vi "Disp3D.vi"(1 "Status":enum16{"In", "Out"}(ring)=enum."Out", 2 "MultR":dbl, 3 "TargXYZ":dbl[](array[numeric])=[0.0, 0.0, 0.0], 4 "PosXYZ":dbl[](array[numeric])=[0.0, 0.0, 0.0], 5 "DrawSize":T1, 6 "Blank":picture) -> (0 "Pic":picture)   [LabVIEW 2013]
uses:
  <vilib>/Utility/miscctls.llb/LVBoundsTypeDef.ctl
panel:
  out "DrawSize 2":T1={"Width"=1662, "Height"=1015}
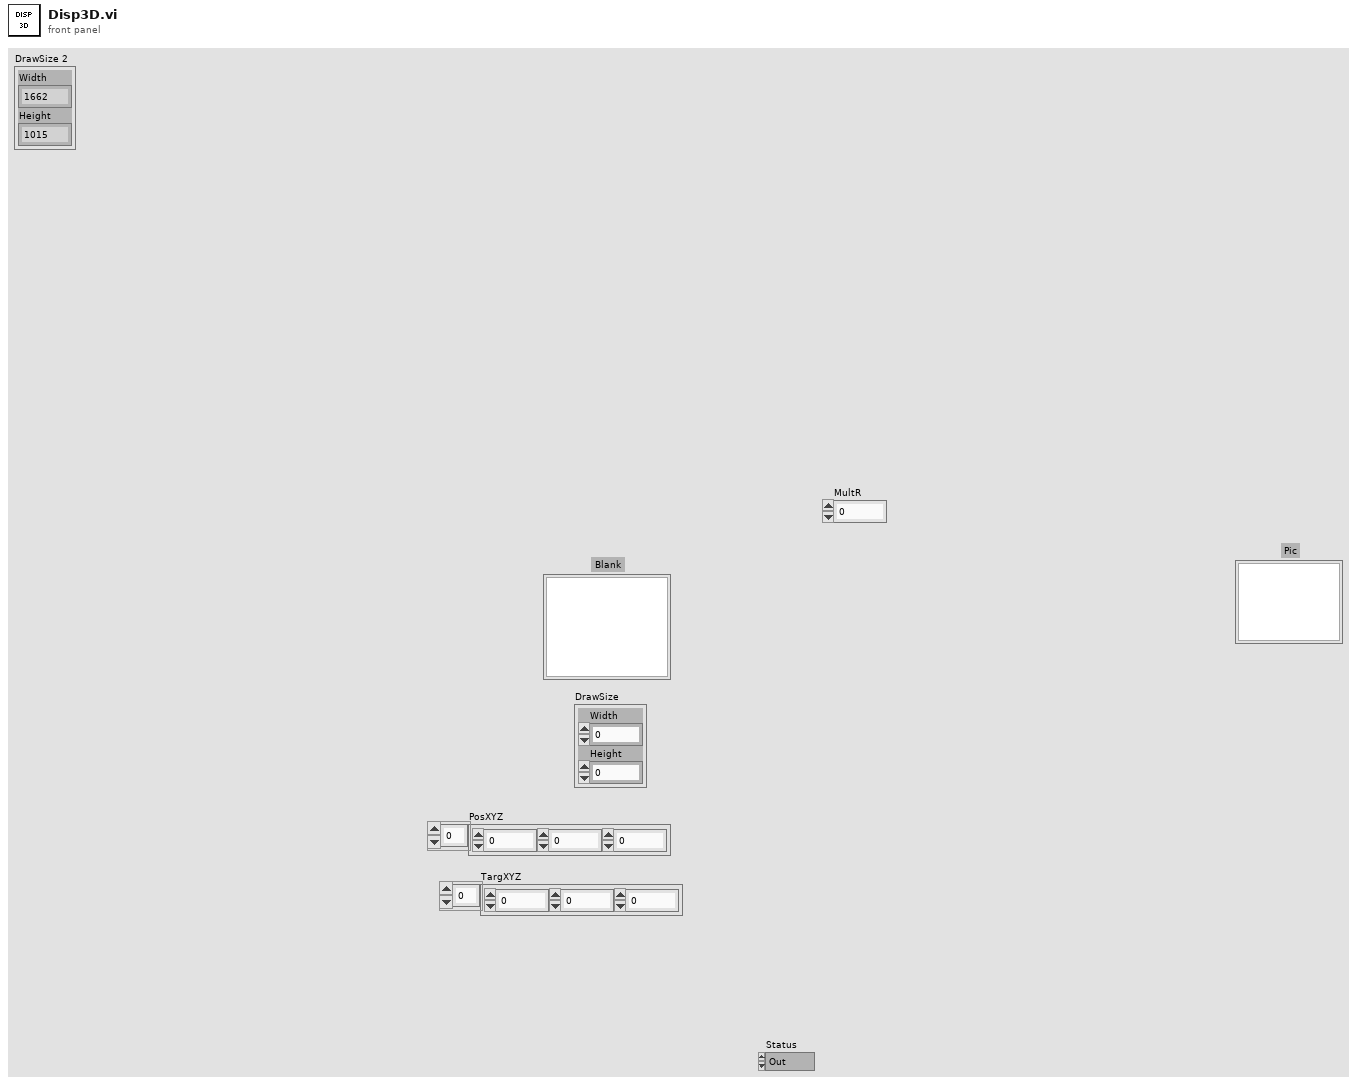
[diagram p1: front panel]
types:
  T1 = typedef "LVBoundsTypeDef.ctl" = cluster{"Width":u32, "Height":u32}
  T2 = cluster{"Width":u16, "Style":enum32{"Solid", "Dash", "Dot", "DashDot", "DashDotDot"}}
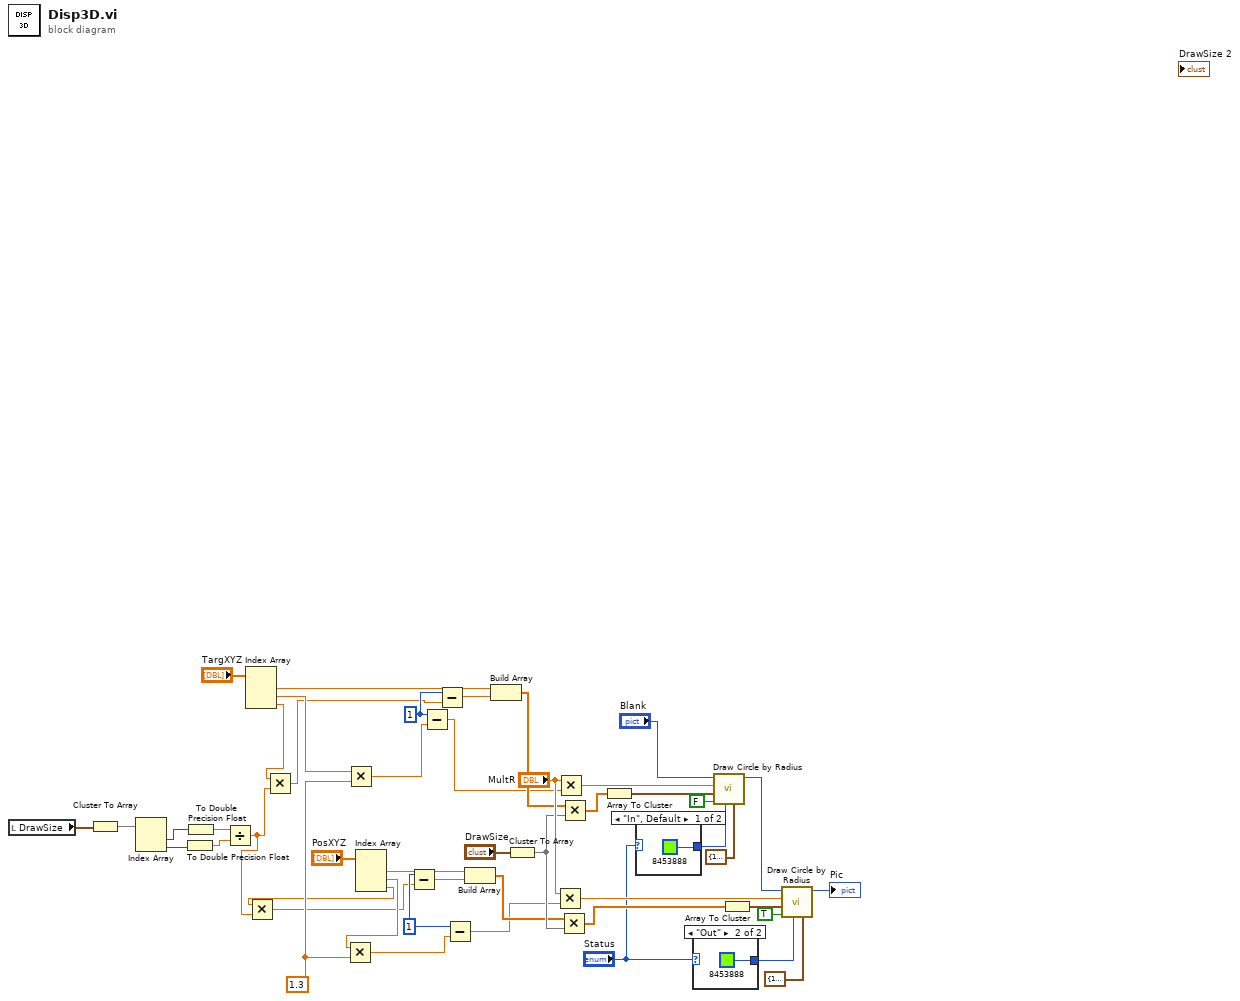
[diagram p0: block diagram]
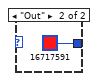
[diagram p2: hidden frame]
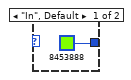
[diagram p3: hidden frame]
diagram:
  w17 = 1.3
  w23 = 1
  w24 = 1
  n1 = local read "DrawSize"() -> (w6:T1)
  n2 = Cluster To Array(cluster=w6) -> (array=w7:u32[])
  n3 = Index Array(array=w7) -> (element #1=w8:u32, element #2=w9:u32)  [unwired: 2 in]
  n4 = To Double Precision Float(number=w9) -> (double precision float=w11:dbl)
  n5 = To Double Precision Float(number=w8) -> (double precision float=w10:dbl)
  n6 = Divide(x=w10, y=w11) -> (x/y=w2:dbl)
  n7 = Index Array(array="TargXYZ") -> (element #1=w21:dbl, element #2=w16:dbl, element #3=w5:dbl)  [unwired: 3 in]
  n8 = Multiply(x=w5, y=w2) -> (x*y=w4:dbl)
  n9 = Multiply(x=w16, y=w17) -> (x*y=w15:dbl)
  n10 = Index Array(array="PosXYZ") -> (element #1=w32:dbl, element #2=w14:dbl, element #3=w3:dbl)  [unwired: 3 in]
  n11 = Multiply(x=w3, y=w2) -> (x*y=w1:dbl)
  n12 = Multiply(x=w14, y=w17) -> (x*y=w18:dbl)
  n13 = Subtract(x=w24, y=w1) -> (x-y=w12:dbl)
  n14 = Subtract(x=w23, y=w15) -> (x-y=w20:dbl)
  n15 = Subtract(x=w23, y=w4) -> (x-y=w13:dbl)
  n16 = Subtract(x=w24, y=w18) -> (x-y=w19:dbl)
  n17 = Build Array(w32, w12) -> (w31:dbl[])
  n18 = Build Array(w21, w13) -> (w22:dbl[])
  n19 = Cluster To Array(cluster="DrawSize") -> (array=w37:u32[])
  n20 = Multiply(x="MultR", y=w19) -> (x*y=w35:dbl)
  n21 = Multiply(x="MultR", y=w20) -> (x*y=w41:dbl)
  n22 = Multiply(x=w31, y=w37) -> (x*y=w39:dbl[])
  n23 = Multiply(x=w22, y=w37) -> (x*y=w43:dbl[])
  n24 = Array To Cluster(array=w43) -> (cluster=w42:cluster{"[0]":dbl, "[1]":dbl})
  n25 = case shown="\"In\", Default" "Status" {
    tunnel: [u32 8453888 u32 16717591] -> w26
    frame "In", Default {
    }
    frame "Out" {
    }
  }
  n26 = case shown="\"Out\"" "Status" {
    tunnel: [u32 8453888 u32 8453888] -> w27
    frame "In", Default {
    }
    frame "Out" {
    }
  }
  n27 = call <vilib>:"Draw Circle by Radius.vi"("pen"=T2 {"Width"=10, "Style"=enum."Solid"}, "color(black)"=w26, "fill?(F)"=FALSE, "pixel center"=w42, "radius"=w41, "picture"="Blank") -> ("new picture"=w47:picture)  [unwired: 5 in]
  n28 = Array To Cluster(array=w39) -> (cluster=w36:cluster{"[0]":dbl, "[1]":dbl})
  n29 = call <vilib>:"Draw Circle by Radius.vi"("pen"=T2 {"Width"=10, "Style"=enum."Solid"}, "color(black)"=w27, "fill?(F)"=TRUE, "pixel center"=w36, "radius"=w35, "picture"=w47) -> ("new picture"=→"Pic":picture)  [unwired: 5 in]
